vi "浊度电极校准.vi"() -> ()   [LabVIEW 2016, in "国弘多参数.lvlib"]
panel:
  out "提示":string
  in  "第二点通过校正":bool
  in  "第一点通过校正":bool
  in  "第二点校正":bool
  in  "第一点校正":bool
  out "标液2":dbl
  out "标液1":dbl
  out "原始读取值":dbl
  out "偏移值补偿":dbl
  out "电极斜率":dbl
  out "电极零点":dbl
  # "浊度电极设定"
  # "NTU"
  # "NTU"
  # "%"
  # "NTU"
  # "电极校正"
  # "标准液值:"
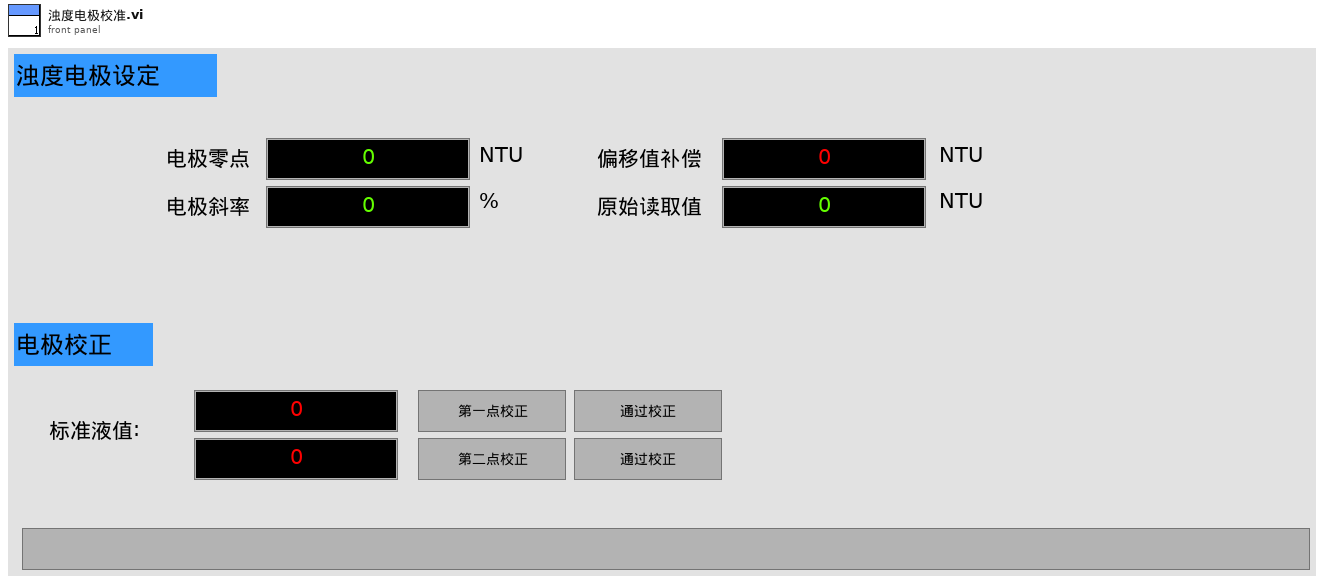
[diagram p1: front panel]
types:
  T1 = cluster{"电极状态标志":u16, "电极型号标志":u16, "浊度测量值":sgl, "温度测量值":sgl, "浊度信号值":sgl, "浊度偏移修正值":sgl, "温度偏移修正值":sgl, "手动温度补偿值":sgl, "浊度电极零点":sgl, "浊度电极斜率":sgl, "第1点标准值记录":sgl, "第1点信号值记录":sgl, "第1点温度值记录":sgl, "第2点标准值记录":sgl, "第2点信号值记录":sgl, "第2点温度值记录":sgl, "命令滤波设定":u16, "温度模式":enum16{"ATC", "MTC"}, "生产批次":u16, "电极序号":u16, "串口地址":u16, "串口波特率":enum16{"9600", "19200", "115200"}, "串口校验位":enum16{"NONE", "ODD", "EVEN"}, "串口停止位":enum16{"1bit", "2bit"}, "第一点标准值":sgl, "第二点标准值":sgl}
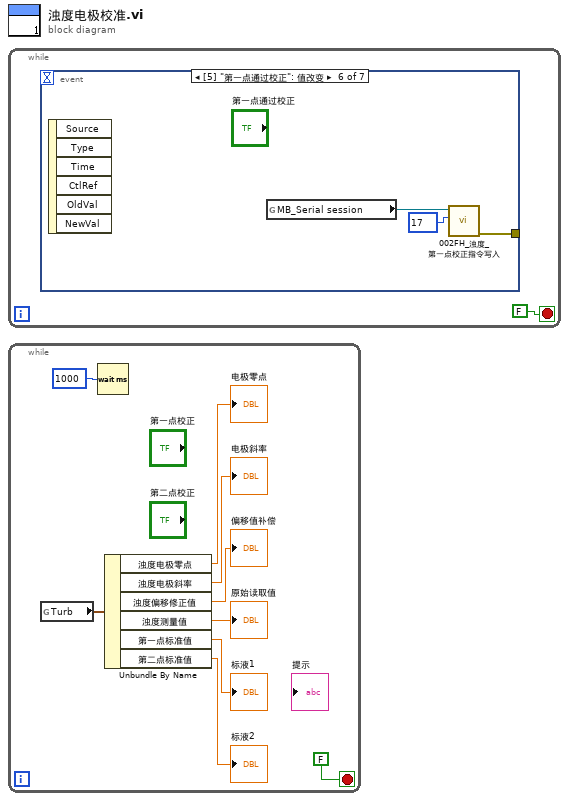
[diagram p0: block diagram]
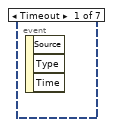
[diagram p2: hidden frame]
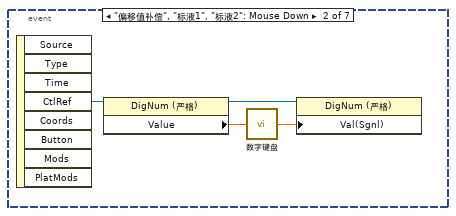
[diagram p3: hidden frame]
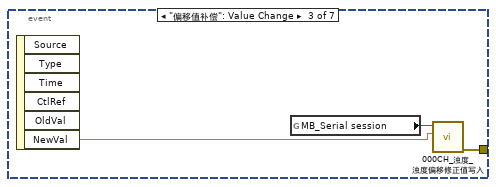
[diagram p4: hidden frame]
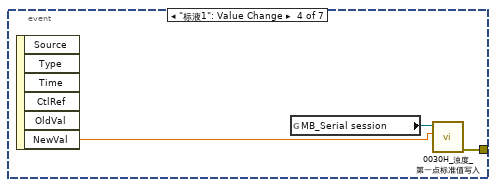
[diagram p5: hidden frame]
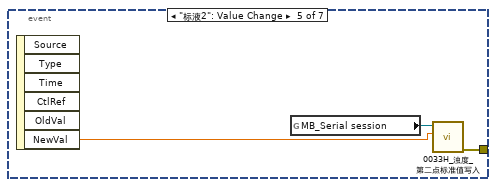
[diagram p6: hidden frame]
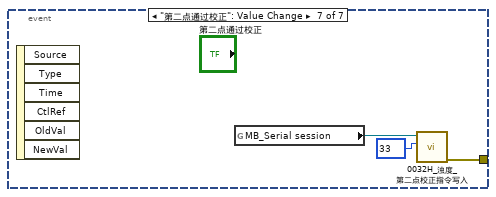
[diagram p7: hidden frame]
diagram:
  n1 = while {
    stop <- FALSE stop-if-true
    n2 = event shown="[5] \"第一点通过校正\": 值改变" {
      selector: _ -> [_ _ _ _ _ _ _]
      dyn-events: _ -> [_ _ _ _ _ _ _]
      timeout: _ -> [_ _ _ _ _ _ _]
      tunnel: [_ _ w6 w9 w13 w17 w20] -> _
      event Timeout {
        n3 = event-data() -> ()  [unwired: 1 in, 3 out]
      }
      event "偏移值补偿", "标液1", "标液2": Mouse Down {
        n4 = event-data() -> ("CtlRef"=w2:refnum<vi>)  [unwired: 1 in, 7 out]
        n5 = property class="DigNum (严格)"(reference=w2) -> (reference out=w3:refnum<vi>, "Value"=w4:dbl)  [unwired: 1 in, 1 out]
        n6 = call "数字键盘.vi"("OldNumber"=w4) -> ("NewNumber"=w5:sgl)
        n7 = property class="DigNum (严格)"(reference=w3, "Val(Sgnl)"=w5) -> ()  [unwired: 1 in, 2 out]
      }
      event "偏移值补偿": Value Change {
        n8 = event-data() -> ("NewVal"=w7:dbl)  [unwired: 1 in, 5 out]
        n9 = global read "过程全局变量.vi" "MB_Serial session"() -> (w8:refnum<class "MB_Master_Serial.lvclass">)
        n10 = call "000CH_浊度_浊度偏移修正值写入.vi"("数值"=w7, "MB_Serial session in"=w8) -> ("error out"=w6:errorcluster)  [unwired: 8 in, 1 out]
      }
      event "标液1": Value Change {
        n11 = event-data() -> ("NewVal"=w11:dbl)  [unwired: 1 in, 5 out]
        n12 = global read "过程全局变量.vi" "MB_Serial session"() -> (w10:refnum<class "MB_Master_Serial.lvclass">)
        n13 = call "0030H_浊度_第一点标准值写入.vi"("数值"=w11, "MB_Serial session in"=w10) -> ("error out"=w9:errorcluster)  [unwired: 8 in, 1 out]
      }
      event "标液2": Value Change {
        n14 = event-data() -> ("NewVal"=w12:dbl)  [unwired: 1 in, 5 out]
        n15 = global read "过程全局变量.vi" "MB_Serial session"() -> (w14:refnum<class "MB_Master_Serial.lvclass">)
        n16 = call "0033H_浊度_第二点标准值写入.vi"("数值"=w12, "MB_Serial session in"=w14) -> ("error out"=w13:errorcluster)  [unwired: 8 in, 1 out]
      }
      event "第一点通过校正": Value Change {
        n17 = event-data() -> ()  [unwired: 1 in, 6 out]
        n18 = global read "过程全局变量.vi" "MB_Serial session"() -> (w16:refnum<class "MB_Master_Serial.lvclass">)
        n19 = call "002FH_浊度_第一点校正指令写入.vi"("数值"=u16 17, "MB_Serial session in"=w16) -> ("error out"=w17:errorcluster)  [unwired: 8 in, 1 out]
      }
      event "第二点通过校正": Value Change {
        n20 = event-data() -> ()  [unwired: 1 in, 6 out]
        n21 = global read "过程全局变量.vi" "MB_Serial session"() -> (w18:refnum<class "MB_Master_Serial.lvclass">)
        n22 = call "0032H_浊度_第二点校正指令写入.vi"("数值"=u16 33, "MB_Serial session in"=w18) -> ("error out"=w20:errorcluster)  [unwired: 8 in, 1 out]
      }
    }
  }
  n23 = while {
    stop <- FALSE stop-if-true
    n24 = global read "过程全局变量.vi" "Turb"() -> (w27:T1)
    n25 = Wait (ms)(milliseconds to wait=u32 1000 ("等待时间（毫秒）")) -> ()  [unwired: 1 out]
    n26 = Unbundle By Name(w27) -> ("浊度电极零点"=→"电极零点":sgl, "浊度电极斜率"=→"电极斜率":sgl, "浊度偏移修正值"=→"偏移值补偿":sgl, "浊度测量值"=→"原始读取值":sgl, "第一点标准值"=→"标液1":sgl, "第二点标准值"=→"标液2":sgl)
  }
